vi "ziExample-Module-Sweeper.vi"() -> ()   [LabVIEW 2016]
doc: "Control a Zurich instrument device via the LabOne Labview API. \nRequirements: Zurich Instruments MFLI, HF2 or UHFLI \nThis example shows how to start a sweeper module and retrieve data.\n\n© Zurich Instruments AG, www.zhinst.com"
uses:
  <instrlib>/Zurich Instruments LabOne/Public/Modules/ziTypeModSweeperImpedanceWave.ctl
  <instrlib>/Zurich Instruments LabOne/Public/Modules/ziTypeModSweeperDemodWave.ctl
  <instrlib>/Zurich Instruments LabOne/Public/Modules/ziTypeModSweeperDoubleWave.ctl
  <instrlib>/Zurich Instruments LabOne/Public/Modules/ziTypeModEnum.ctl
  <instrlib>/Zurich Instruments LabOne/Public/Configure/ziSetValueDoubleArray.vi
  <instrlib>/Zurich Instruments LabOne/Public/Modules/ziModSetValueBinary.vi
  <instrlib>/Zurich Instruments LabOne/Public/Modules/ziModSetValueDoubleArray.vi
  <instrlib>/Zurich Instruments LabOne/Public/Modules/ziModSetValueDouble.vi
  <instrlib>/Zurich Instruments LabOne/Public/Modules/ziModGetDoubleData.vi
  <instrlib>/Zurich Instruments LabOne/Public/Modules/ziModGetSweeperData.vi
  <instrlib>/Zurich Instruments LabOne/Zurich Instruments LabOne.lvlib
panel:
  in  "Samplecount":dbl=100.0
  in  "Stop":dbl=70000000.0
  in  "Start":dbl=40000000.0
  in  "Gridnode":string="oscs/0/freq"
  out "SweeperDoubleWaveArray":T1[](array[typedef]) {"bandwidthMode" format="%f"; "flags" format="%f"; "sampleFormat" format="%f"; "sweepMode" format="%f"; "sampleCount" format="%f"; "timestamp" format="%f"}
  out "SweeperDemodWaveArray":T2[](array[typedef]) {"bandwidthMode" format="%f"; "flags" format="%f"; "sampleFormat" format="%f"; "sweepMode" format="%f"; "sampleCount" format="%f"; "timestamp" format="%f"}
  out "SweeperImpedanceWaveArray":T3[](array[typedef]) {"bandwidthMode" format="%f"; "flags" format="%f"; "sampleFormat" format="%f"; "sweepMode" format="%f"; "sampleCount" format="%f"; "timestamp" format="%f"}
  out "Error Out":errorcluster
  in  "Address":string="DEV2090"
  out "Settings":T4
  out "Selected Device":string="DEV2090"
  in  "subscribepath":string="demods/0/sample" caption="Subscribe Path"
  out "Sweeper Phase":cluster{"grid":dbl[], "r_avg":dbl[]}(graph)
  out "Sweeper R":cluster{"grid":dbl[], "value":dbl[]}[](graph)
  # "ziExample-SweepModul.vi\nRequirements: HF2LI, UHFLI or MFLI\nsee block diagram for VI description"
  # "Tested Devices:\n- HF2LI\n- UHFLI\n- MFLI"
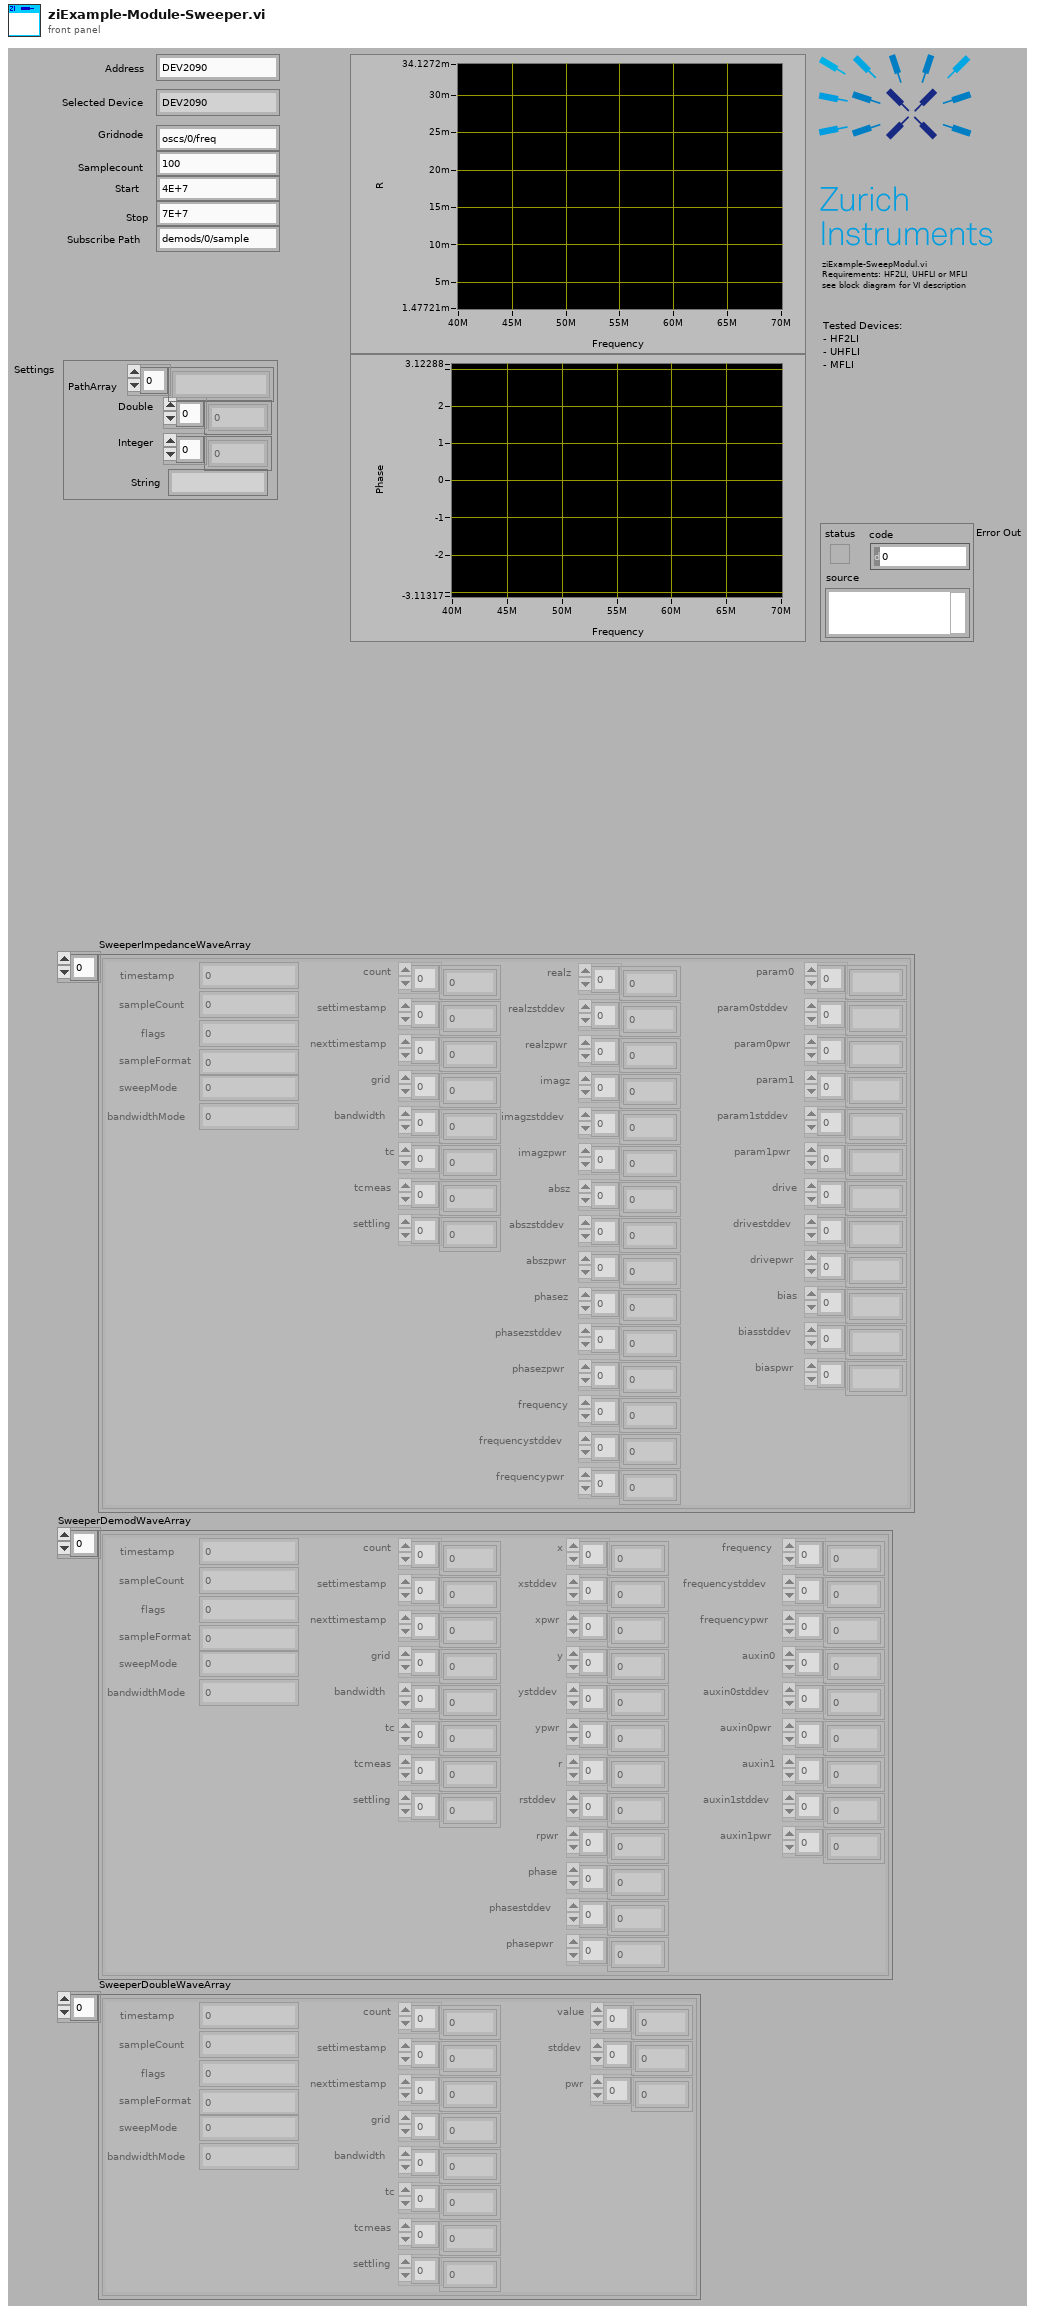
[diagram p1: front panel]
types:
  T1 = typedef "Zurich Instruments LabOne.lvlib/ziTypeModSweeperDoubleWave.ctl" = cluster{"timestamp":u64, "sampleCount":u64, "flags":u8, "sampleFormat":u8, "sweepMode":u8, "bandwidthMode":u8, "count":u64[], "settimestamp":u64[], "nexttimestamp":u64[], "grid":dbl[], "bandwidth":dbl[], "tc":dbl[], "tcmeas":dbl[], "settling":dbl[], "value":dbl[], "stddev":dbl[], "pwr":dbl[]}
  T2 = typedef "Zurich Instruments LabOne.lvlib/ziTypeModSweeperDemodWave.ctl" = cluster{"timestamp":u64, "sampleCount":u64, "flags":u8, "sampleFormat":u8, "sweepMode":u8, "bandwidthMode":u8, "count":u64[], "settimestamp":u64[], "nexttimestamp":u64[], "grid":dbl[], "bandwidth":dbl[], "tc":dbl[], "tcmeas":dbl[], "settling":dbl[], "x":dbl[], "xstddev":dbl[], "xpwr":dbl[], "y":dbl[], "ystddev":dbl[], "ypwr":dbl[], "r":dbl[], "rstddev":dbl[], "rpwr":dbl[], "phase":dbl[], "phasestddev":dbl[], "phasepwr":dbl[], "frequency":dbl[], "frequencystddev":dbl[], "frequencypwr":dbl[], "auxin0":dbl[], "auxin0stddev":dbl[], "auxin0pwr":dbl[], "auxin1":dbl[], "auxin1stddev":dbl[], "auxin1pwr":dbl[]}
  T3 = typedef "Zurich Instruments LabOne.lvlib/ziTypeModSweeperImpedanceWave.ctl" = cluster{"timestamp":u64, "sampleCount":u64, "flags":u8, "sampleFormat":u8, "sweepMode":u8, "bandwidthMode":u8, "count":u64[], "settimestamp":u64[], "nexttimestamp":u64[], "grid":dbl[], "bandwidth":dbl[], "tc":dbl[], "tcmeas":dbl[], "settling":dbl[], "realz":dbl[], "realzstddev":dbl[], "realzpwr":dbl[], "imagz":dbl[], "imagzstddev":dbl[], "imagzpwr":dbl[], "absz":dbl[], "abszstddev":dbl[], "abszpwr":dbl[], "phasez":dbl[], "phasezstddev":dbl[], "phasezpwr":dbl[], "frequency":dbl[], "frequencystddev":dbl[], "frequencypwr":dbl[], "param0":dbl[], "param0stddev":dbl[], "param0pwr":dbl[], "param1":dbl[], "param1stddev":dbl[], "param1pwr":dbl[], "drive":dbl[], "drivestddev":dbl[], "drivepwr":dbl[], "bias":dbl[], "biasstddev":dbl[], "biaspwr":dbl[]}
  T4 = cluster{"String":string, "Integer":dbl[], "Double":dbl[], "PathArray":string[]}
  T5 = typedef "Zurich Instruments LabOne.lvlib/ziTypeModEnum.ctl" = u16
  T6 = typedef "Zurich Instruments LabOne.lvlib/ziTypeHandle.ctl" = cluster{"handleValid":bool, "Conn":u64, "Path Prefix":string, "Handle":u64, "Connected":bool, "Clockbase(s)":dbl}
  T7 = typedef "Zurich Instruments LabOne.lvlib/ziTypeModHandle.ctl" = cluster{"handleValid":bool, "Conn":u64, "ModHandle":u64, "moduleID":string, "Path Prefix":string}
  T8 = cluster{"String":string, "Integer":i64[], "Double":dbl[], "PathArray":string[]}
  T9 = typedef "Zurich Instruments LabOne.lvlib/ziTypeModResults.ctl" = cluster{"PathArray":string[], "ValueType":T10, "NoOfResults":u64, "ziGenericHeader":T11[]}
  T10 = typedef "Zurich Instruments LabOne.lvlib/ziTypePollType.ctl" = enum16{"NONE", "DOUBLE_DATA", "INTEGER_DATA", "DEMOD_SAMPLE", "SCOPE_WAVE_HF2", "AUXIN_SAMPLE", "DIO_SAMPLE", "BYTE_ARRAY", "PWA_WAVE", "9", "10", "11", "12", "13", "14", "15", "TREE_CHANGE_DEPRI", "17", "ERROR", "19", "20", "21", "22", "23", "24", "25", "26", "27", "28", "29", "30", "31", "DOUBLE_DATA_TS", "INTEGER_DATA_TS", "34", "SCOPE_WAVE", "SCOPE_WAVE_EX", "37", "BYTE_ARRAY_TS", "39", "40", "41", "42", "43", "44", "45", "CNT_DATA", "47", "TREE_CHANGE", "49", "50", "51", "52", "53", "54", "55", "56", "57", "58", "59", "60", "61", "62", "63", "SWEEPER_DATA", "SPECTRUM_DATA", "ADVISOR_DATA", "VECTOR_DATA", "IMP_DATA"}
  T11 = typedef "Zurich Instruments LabOne.lvlib/ziTypeModGenericHeader.ctl" = cluster{"HeaderType":enum8{"HEADER_TYPE_NONE", "HEADER_TYPE_SWTRIGGER", "HEADER_TYPE_SWEEPER"}, "SampleFormat":u8, "SystemTime":timestamp, "CreatedTimeStamp":u64, "ChangedTimeStamp":u64, "Flags":u32, "ChunkSizeBytes":u64, "Name":string, "Status":u32, "GroupIndex":u32, "Color":u32, "ActiveRow":u32, "TriggerNumber":u64, "GridRows":u32, "GridCols":u32, "GridMode":u32, "GridOperation":u32, "GridDirection":u32, "GridRepetitions":u32, "GridColDelta":dbl, "GridColOffset":dbl, "GridRowDelta":dbl, "GridRowOffset":dbl, "Bandwidth":dbl, "Center":dbl, "Nenbw":dbl}
  T12 = typedef "Zurich Instruments LabOne.lvlib/ziTypeDoubleDataTS.ctl" = cluster{"Timestamp (ticks)":u64[], "Value":dbl[]}
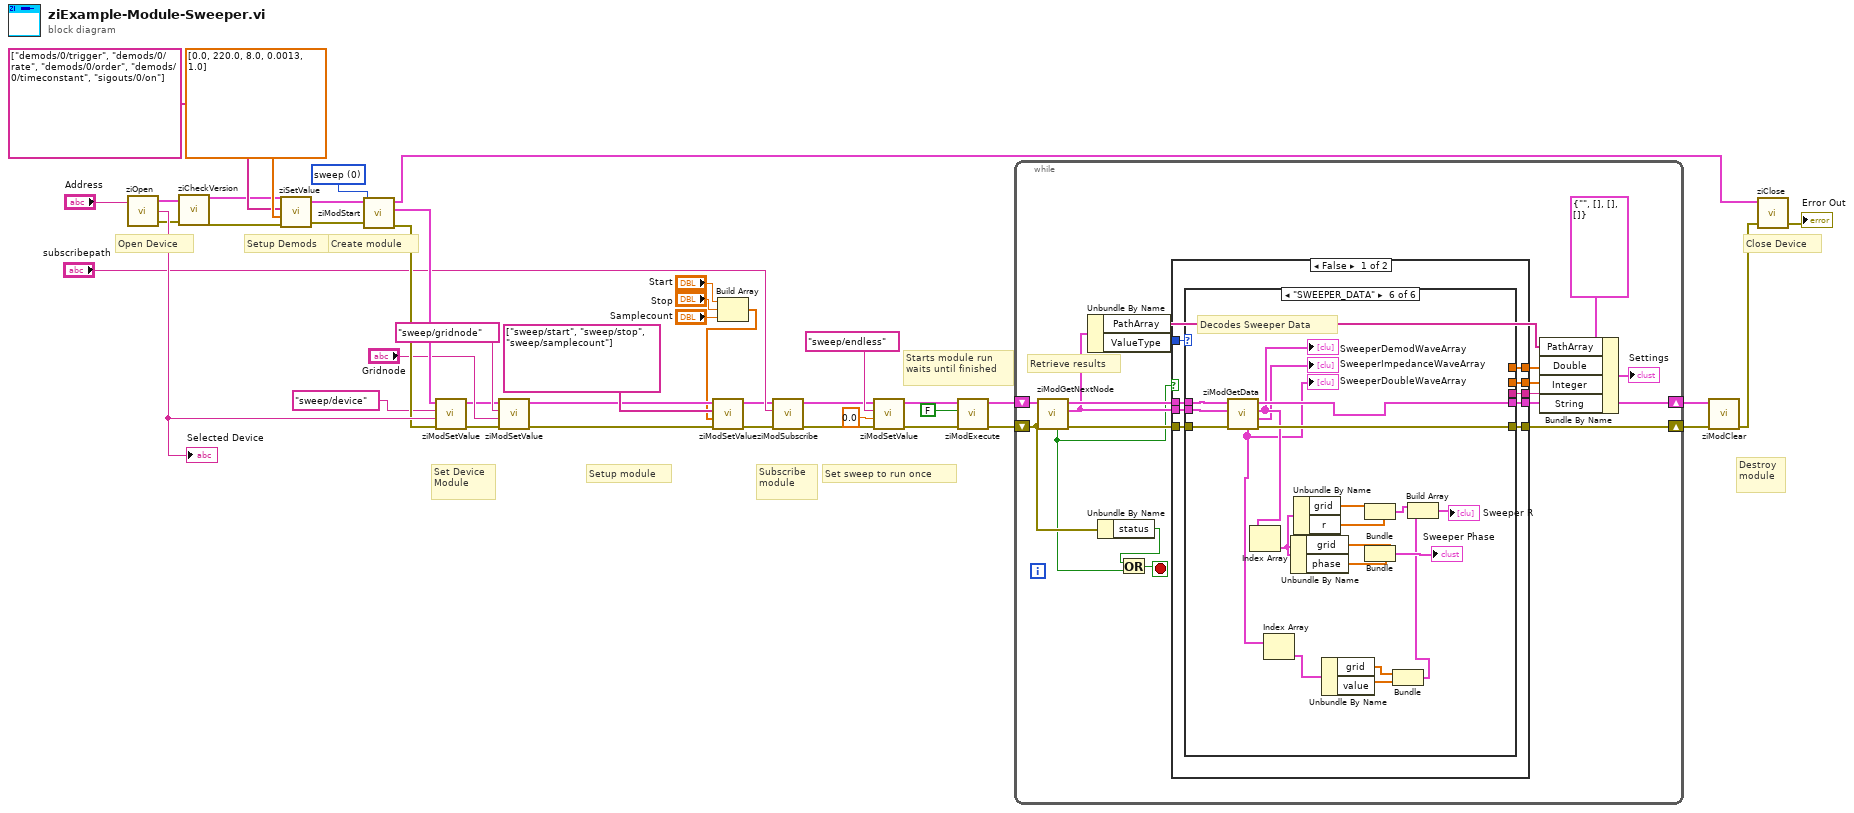
[diagram p0: block diagram]
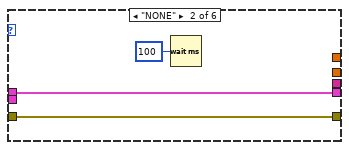
[diagram p3: hidden frame]
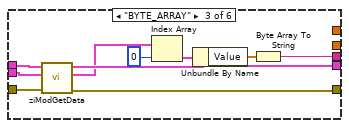
[diagram p4: hidden frame]
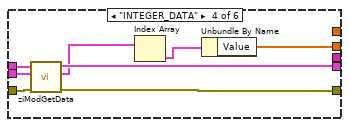
[diagram p5: hidden frame]
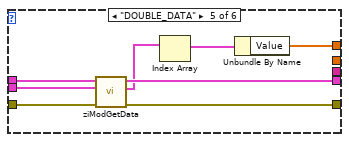
[diagram p6: hidden frame]
diagram:
  w1 = T5 0 items=["sweep", "scopeModule", "dataAcquisitionModule", "pidAdvisor", "awgModule", "impedanceModule", "multiDeviceSyncModule", "zoomFFT", "trigger", "deviceSettings", "record"] ("module Id")
  # "Setup Demods"
  # "Set Device\nModule"
  # "Destroy\nmodule"
  # "Starts module run\nwaits until finished"
  # "Set sweep to run once"
  # "Subscribe\nmodule"
  # "Setup module"
  # "Create module"
  # "Close Device"
  # "Open Device"
  n1 = call <instrlib>:"ziOpen.vi"("Address"="Address") -> ("Error Out"=w4:errorcluster, "Selected Device"=w41:string, "HandleOut"=w5:T6)  [unwired: 1 in, 2 out]
  "Selected Device" <- w41
  n2 = call <instrlib>:"ziCheckVersion.vi"("Handle In"=w5, "Error In"=w4) -> ("Handle Out"=w2:T6, "Error Out"=w3:errorcluster)  [unwired: 11 in, 1 out]
  n3 = call-poly <instrlib>:"ziSetValue.vi"("Error In"=w3, "Values"=dbl[] [0.0, 220.0, 8.0, 0.0013, 1.0], "Paths"=string[] ["demods/0/trigger", "demods/0/rate", "demods/0/order", "demods/0/timeconstant", "sigouts/0/on"], "Handle In"=w2) -> ("Error Out"=w27:errorcluster, "Handle Out"=w28:T6)  [unwired: 1 in]
  n4 = call <instrlib>:"ziModStart.vi"("Error In"=w27, "module Id"=w1, "Handle In"=w28) -> ("Error Out"=w30:errorcluster, "ModHandle Out"=w31:T7, "Handle Out"=w40:T6)  [unwired: 6 in]
  n5 = call-poly <instrlib>:"ziModSetValue.vi"("Error In"=w30, "Data"=w41, "Path"="sweep/device", "ModHandle In"=w31) -> ("Error Out"=w10:errorcluster, "ModHandle Out"=w13:T7)  [unwired: 6 in]
  n6 = call-poly <instrlib>:"ziModSetValue.vi"("Error In"=w10, "Data"="Gridnode", "Path"="sweep/gridnode", "ModHandle In"=w13) -> ("Error Out"=w11:errorcluster, "ModHandle Out"=w12:T7)  [unwired: 6 in]
  n7 = Build Array("Start", "Stop", "Samplecount") -> (w6:dbl[])
  n8 = call-poly <instrlib>:"ziModSetValue.vi"("Error In"=w11, "Values"=w6, "Paths"=string[] ["sweep/start", "sweep/stop", "sweep/samplecount"], "ModHandle In"=w12) -> ("Error Out"=w14:errorcluster, "ModHandle Out"=w15:T7)  [unwired: 6 in]
  n9 = call <instrlib>:"ziModSubscribe.vi"("Error In"=w14, "Path"="subscribepath", "ModHandle In"=w15) -> ("Error Out"=w37:errorcluster, "ModHandle Out"=w38:T7)  [unwired: 6 in]
  n10 = call-poly <instrlib>:"ziModSetValue.vi"("Error In"=w37, "Value"=0.0, "Path"="sweep/endless", "ModHandle In"=w38) -> ("Error Out"=w36:errorcluster, "ModHandle Out"=w35:T7)  [unwired: 6 in]
  n11 = call <instrlib>:"ziModExecute.vi"("Error In"=w36, "Modal (F)"=FALSE ("Modal"), "ziModHandle In"=w35) -> ("Error Out"=w32:errorcluster, "ziModHandle Out"=w34:T7)  [unwired: 5 in, 1 out]
  n12 = while {
    shift-right: [w57] -> w17
    shift-left: w34 -> [w59]
    shift-right: [w56] -> w18
    shift-left: w32 -> [w45]
    stop <- w44 stop-if-true
    # "Retrieve results"
    n13 = call <instrlib>:"ziModGetNextNode.vi"("Error In"=w45, "ModHandle In"=w59) -> ("Error Out"=w55:errorcluster, "ModResults"=w47:T9, "ModHandle Out"=w58:T7, "NoData"=w43:bool)  [unwired: 6 in]
    n14 = Unbundle By Name(w47) -> ("PathArray"=w49:string[], "ValueType"=w48:T10)
    n15 = Unbundle By Name(w45) -> ("status"=w46:bool)
    n16 = Or(x=w46, y=w43) -> (x .or. y?=w44:bool)
    n17 = case shown="False" w43 {
      tunnel: w58 -> [w68 w120]
      tunnel: [w67 w120] -> w57
      tunnel: [w66 w121] -> w56
      tunnel: w55 -> [w65 w121]
      tunnel: w47 -> [w64 _]
      tunnel: [w63 _] -> w54
      tunnel: [w62 _] -> w53
      tunnel: [w61 _] -> w52
      tunnel: w48 -> [w60 _]
      frame False {
        n18 = case shown="\"SWEEPER_DATA\"" w60 {
          tunnel: w68 -> [w70 w73 w83 w91 w99 w109]
          tunnel: w64 -> [_ _ w82 w90 w98 w119]
          tunnel: w65 -> [w69 w72 w81 w89 w97 w118]
          tunnel: [w69 w72 w80 w88 w95 w117] -> w66
          tunnel: [w70 w73 w79 w87 w96 w116] -> w67
          tunnel: [_ _ w74 _ _ _] -> w63
          tunnel: [_ _ _ w86 _ _] -> w62
          tunnel: [_ _ _ _ w94 _] -> w61
          frame Default {
          }
          frame "NONE" {
            n19 = Wait (ms)(milliseconds to wait=u32 100) -> ()  [unwired: 1 out]
          }
          frame "BYTE_ARRAY" {
            n20 = call-poly <instrlib>:"ziModGetData.vi"("Error In"=w81, "ModResults"=w82, "ModHandle In"=w83) -> ("Error Out"=w80:errorcluster, "DoubleSample"=w77:T12[], "ModHandle Out"=w79:T7)  [unwired: 4 in, 2 out]
            n21 = Index Array(array=w77, index=0) -> (element=w76:T12)
            n22 = Unbundle By Name(w76) -> ("Value"=w75:dbl[])
            n23 = Byte Array To String(unsigned byte array=w75) -> (string=w74:string)
          }
          frame "INTEGER_DATA" {
            n24 = call-poly <instrlib>:"ziModGetData.vi"("Error In"=w89, "ModResults"=w90, "ModHandle In"=w91) -> ("Error Out"=w88:errorcluster, "DoubleSample"=w85:T12[], "ModHandle Out"=w87:T7)  [unwired: 4 in, 2 out]
            n25 = Index Array(array=w85) -> (element=w84:T12)  [unwired: 1 in]
            n26 = Unbundle By Name(w84) -> ("Value"=w86:dbl[])
          }
          frame "DOUBLE_DATA" {
            n27 = call-poly <instrlib>:"ziModGetData.vi"("Error In"=w97, "ModResults"=w98, "ModHandle In"=w99) -> ("Error Out"=w95:errorcluster, "DoubleSample"=w93:T12[], "ModHandle Out"=w96:T7)  [unwired: 4 in, 2 out]
            n28 = Index Array(array=w93) -> (element=w92:T12)  [unwired: 1 in]
            n29 = Unbundle By Name(w92) -> ("Value"=w94:dbl[])
          }
          frame "SWEEPER_DATA" {
            # "Decodes Sweeper Data"
            n30 = call-poly <instrlib>:"ziModGetData.vi"("Error In"=w118, "ModResults"=w119, "ModHandle In"=w109) -> ("Error Out"=w117:errorcluster, "SweeperImpedanceWaveArray"=→"SweeperImpedanceWaveArray":T3[], "SweeperDemodWaveArray"=w108:T2[], "ModHandle Out"=w116:T7, "SweeperDoubleWaveArray"=w106:T1[])  [unwired: 4 in]
            "SweeperDemodWaveArray" <- w108
            "SweeperDoubleWaveArray" <- w106
            n31 = Index Array(array=w108) -> (element=w110:T2)  [unwired: 1 in]
            n32 = Index Array(array=w106) -> (element=w107:T1)  [unwired: 1 in]
            n33 = Unbundle By Name(w110) -> ("grid"=w112:dbl[], "phase"=w113:dbl[])
            n34 = Unbundle By Name(w110) -> ("grid"=w114:dbl[], "r"=w115:dbl[])
            n35 = Unbundle By Name(w107) -> ("grid"=w105:dbl[], "value"=w104:dbl[])
            n36 = Bundle("grid"=w114, "r"=w115) -> (w101:cluster{"grid":dbl[], "r":dbl[]})  [unwired: 1 in]
            n37 = Bundle("grid"=w112, "phase"=w113) -> (→"Sweeper Phase":cluster{"grid":dbl[], "phase":dbl[]})  [unwired: 1 in]
            n38 = Bundle("grid"=w105, "value"=w104) -> (w102:cluster{"grid":dbl[], "value":dbl[]})  [unwired: 1 in]
            n39 = Build Array(w101, w102) -> (→"Sweeper R":cluster{"grid":dbl[], "value":dbl[]}[])
          }
        }
      }
      frame True {
      }
    }
    n40 = Bundle By Name(cluster=T8 {"String"="", "Integer"=[], "Double"=[], "PathArray"=[]} ("Settings 2"), "PathArray"=w49, "Double"=w52, "Integer"=w53, "String"=w54) -> (→"Settings":T8)
  }
  n41 = call <instrlib>:"ziModClear.vi"("Error In"=w18, "ziModHandle In"=w17) -> ("Error Out"=w42:errorcluster)  [unwired: 7 in, 1 out]
  n42 = call <instrlib>:"ziClose.vi"("Error In"=w42, "Handle In"=w40) -> ("Error Out"=→"Error Out":errorcluster)  [unwired: 2 in, 1 out]
